vi "NF LI56xx dvr FREQuency psd1 SMULtiplier.vi"(8 "error in":errorcluster caption="error in (no error)" {"code" format="%.0x"}, 9 "Read(F)":bool, 10 "set subharmonic order":u8=1 min=1 max=63 step=1, 11 "VISA resource name":refnum<visa-resource-name>) -> (0 "error out":errorcluster {"code" format="%.0x"}, 2 "query subharmonic order":string, 3 "VISA resource name copy":refnum<visa-resource-name>)   [LabVIEW 2019]
doc: "Sets/queries the subharmonic order m for measurement (primary PSD). \nThe signal that is 1/m-th the reference signal can be measured. \nHarmonics measurement must be enabled with the [:SENSe]:FREQuency[1]:HARMonics ON command."
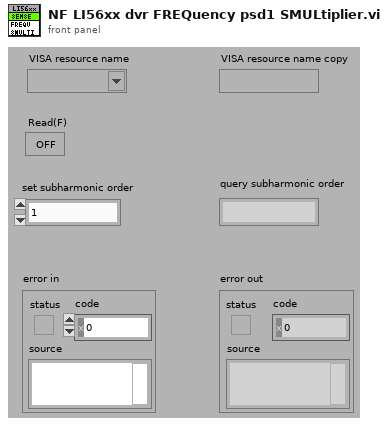
[diagram p1: front panel]
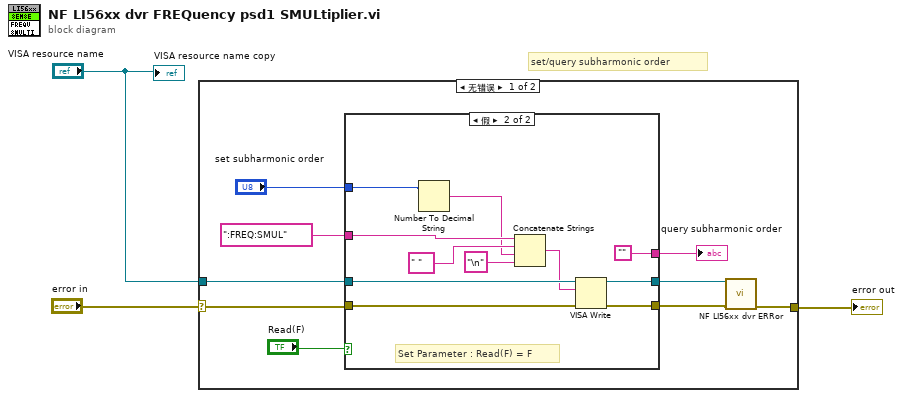
[diagram p0: block diagram]
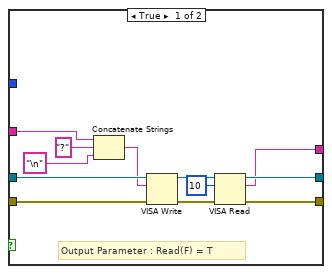
[diagram p2: hidden frame]
diagram:
  # "set/query subharmonic order"
  n1 = case shown="无错误" "error in" {
    selector: "error in" -> [w11 w36]
    tunnel: [w5 w36] -> w3
    tunnel: "VISA resource name" -> [w10 _]
    frame No Error {
      n2 = case shown="假" "Read(F)" {
        tunnel: w10 -> [w24 w35]
        tunnel: [w21 w32] -> w7
        tunnel: [w20 w33] -> w6
        tunnel: w11 -> [w19 w34]
        tunnel: [w15 ""] -> w9
        tunnel: "set subharmonic order" -> [_ w26]
        tunnel: ":FREQ:SMUL" ("•¶Žš—ñ") -> [w13 w27]
        frame True {
          # "Output Parameter : Read(F) = T"
          n3 = Concatenate Strings(w13, "?" ("Œ`Ž®•¶Žš—ñ"), "\n" ("Œ`Ž®•¶Žš—ñ")) -> (w16:string)
          n4 = VISA Write(VISA resource name=w24, write buffer=w16, error in (no error)=w19) -> (VISA resource name out=w22:refnum<visa-resource-name>, error out=w23:errorcluster)  [unwired: 1 out]
          n5 = VISA Read(VISA resource name=w22, byte count=u32 10 ("バイトカウント（0）"), error in (no error)=w23) -> (VISA resource name out=w21:refnum<visa-resource-name>, read buffer=w15:string, error out=w20:errorcluster)  [unwired: 1 out]
        }
        frame False {
          # "Set Parameter : Read(F) = F"
          n6 = Number To Decimal String(number=w26) -> (decimal integer string=w25:string)  [unwired: 1 in]
          n7 = Concatenate Strings(w27, " ", w25, "\n" ("Œ`Ž®•¶Žš—ñ")) -> (w30:string)
          n8 = VISA Write(VISA resource name=w35, write buffer=w30, error in (no error)=w34) -> (VISA resource name out=w32:refnum<visa-resource-name>, error out=w33:errorcluster)  [unwired: 1 out]
        }
      }
      "query subharmonic order" <- w9
      n9 = call "NF LI56xx dvr ERRor.vi"("VISA resource name"=w7, "error in (no error)"=w6) -> ("error out"=w5:errorcluster)  [unwired: 10 in, 3 out]
    }
    frame Error {
    }
  }
  "error out" <- w3
  "VISA resource name copy" <- "VISA resource name"
